vi "HeaderuRayon.vi"(1 "UUT":string, 2 "S/N":string, 3 "Oper.":string) -> (0 "HEADER1":string)   [LabVIEW 2017]
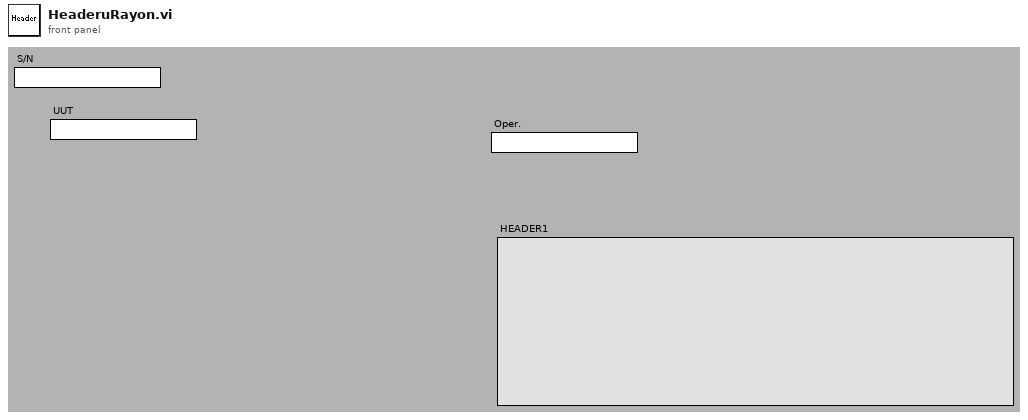
[diagram p1: front panel]
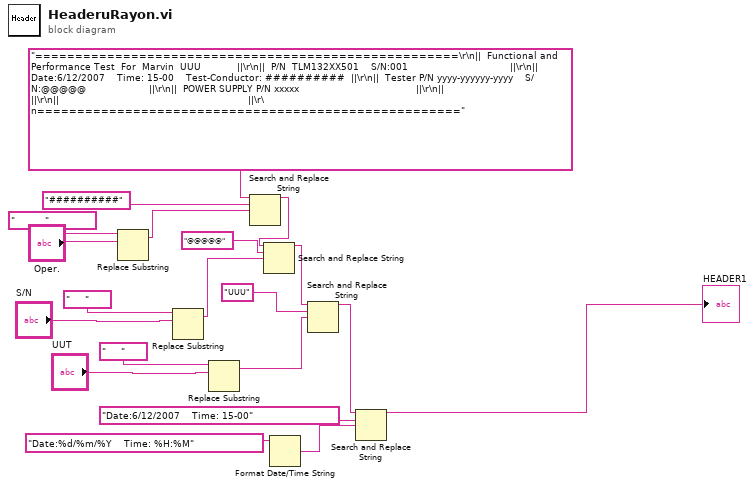
[diagram p0: block diagram]
diagram:
  n1 = Replace Substring(4:"Oper.", 5:"          " ("source")) -> (1:w12:string)  [unwired: 2 in, 1 out]
  n2 = Replace Substring(4:"S/N", 5:"     " ("source")) -> (1:w16:string)  [unwired: 2 in, 1 out]
  n3 = Replace Substring(4:"UUT", 5:"     " ("source")) -> (1:w1:string)  [unwired: 2 in, 1 out]
  n4 = Search and Replace String(input string="=====================================================\r\n||  Functional and Performance Test  For  Marvin  UUU            ||\r\n||  P/N  TLM132XX501    S/N:001                                  ||\r\n||  Date:6/12/2007    Time: 15-00    Test-Conductor: ##########  ||\r\n||  Tester P/N yyyy-yyyyyy-yyyy    S/N:@@@@@                     ||\r\n||  POWER SUPPLY P/N xxxxx                                       ||\r\n||                                                               ||\r\n||                                                               ||\r\n=====================================================" ("source"), search string="##########" ("source"), replace string=w12) -> (result string=w13:string)  [unwired: 5 in, 3 out]
  n5 = Search and Replace String(input string=w13, search string="@@@@@" ("source"), replace string=w16) -> (result string=w3:string)  [unwired: 5 in, 3 out]
  n6 = Format Date/Time String(time format string (%c)="Date:%d/%m/%Y    Time: %H:%M") -> (date/time string=w18:string)  [unwired: 2 in]
  n7 = Search and Replace String(input string=w3, search string="UUU" ("source"), replace string=w1) -> (result string=w4:string)  [unwired: 5 in, 3 out]
  n8 = Search and Replace String(input string=w4, search string="Date:6/12/2007    Time: 15-00" ("time format string (%c)"), replace string=w18) -> (result string=→"HEADER1":string)  [unwired: 5 in, 3 out]
